vi "JKISM+ State Machine Steps Executed on Sub-Module.vi"() -> ()   [LabVIEW 2014]
uses:
  user.lib/_NEVSTOP/JKI State Machine ++/_Support/JKISMQ/_JKISMQFGV.vi
  user.lib/_NEVSTOP/JKI State Machine ++/JKI-State-Machine-Plus.lvlib
panel:
  in  "Exit":bool
  in  "Run":bool
  out "State History of Sub-Module":string
  out "State History of Main":string
  # "SM: Step1\nSM: Step2 @ Sub-Module\nSM: Step3\nSM: Step4 @ Sub-Module\nSM: Event Check"
  # "(back to step1)"
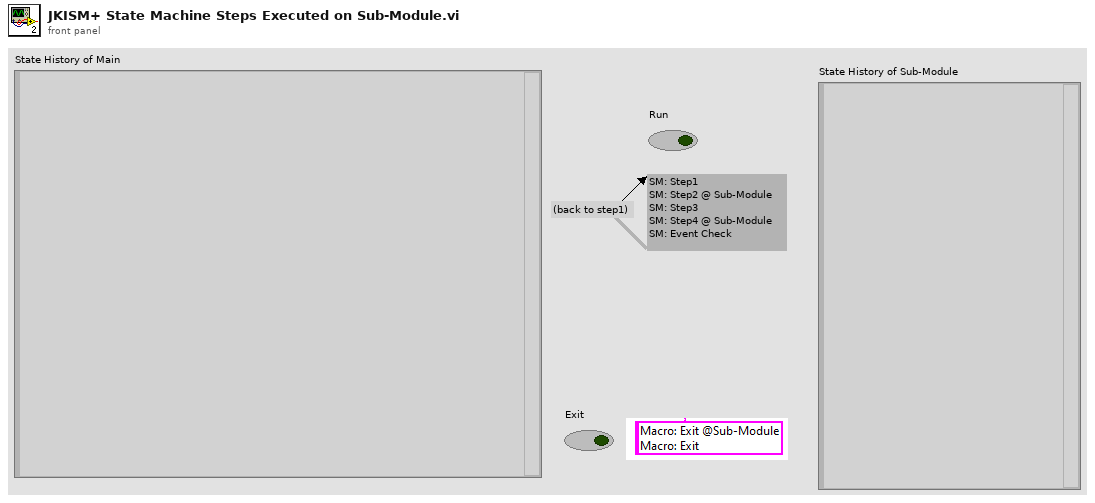
[diagram p1: front panel]
types:
  T1 = enum32{"Invalid", "Standard", "Closed", "Hidden", "Minimized", "Maximized"}
  T2 = enum32{"invalid app kind", "Development System", "Run Time System", "Student Edition", "Embedded LabVIEW", "Evaluation", "Custom"}
  T3 = cluster{"Core":cluster{"Current VI Reference":refnum<vi>, "Close Panel on Exit?":bool}, "Your Boolean data":bool, "State":string}
  T4 = cluster{"Current VI Reference":refnum<vi>, "Close Panel on Exit?":bool}
  T5 = cluster{"Core":cluster{"Current VI Reference":refnum<vi>, "Close Panel on Exit?":bool}, "Your Boolean data":bool, "Your string data":string}
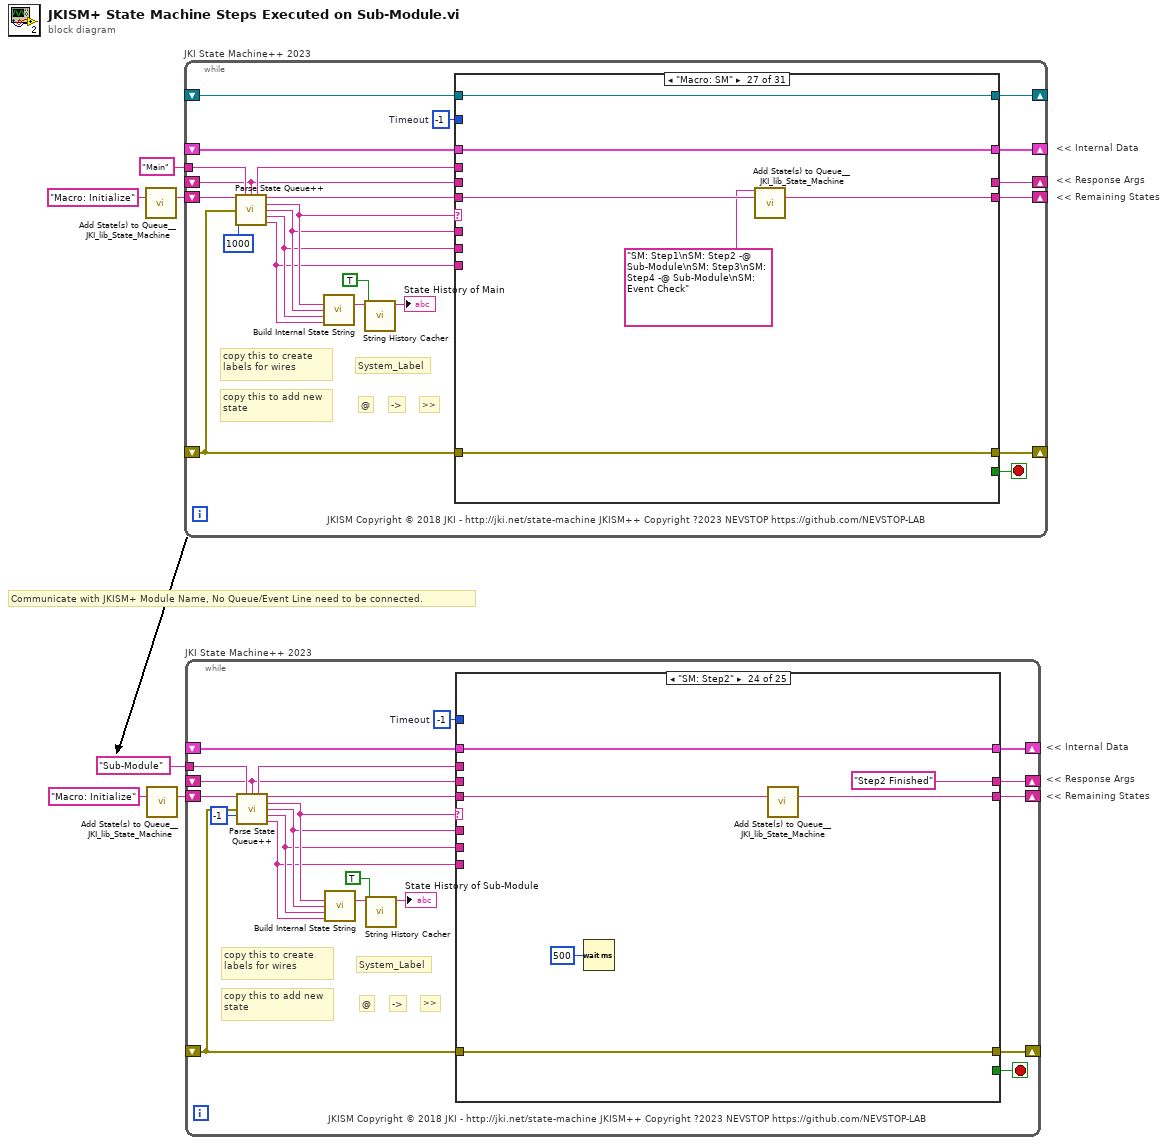
[diagram p0: block diagram]
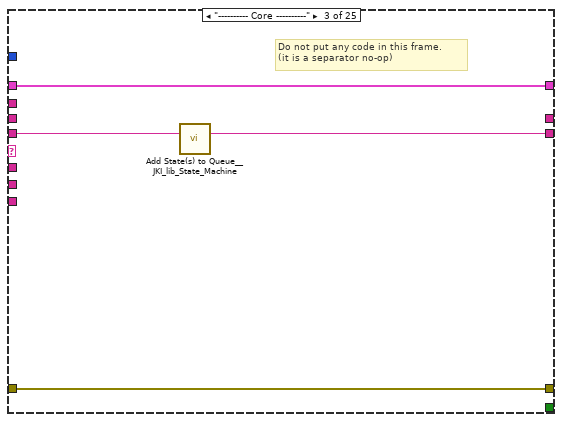
[diagram p4: hidden frame]
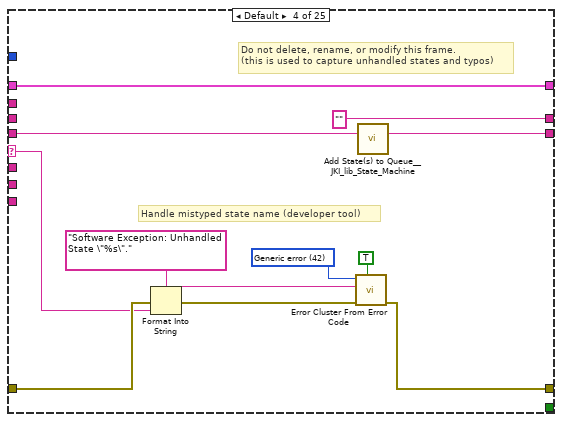
[diagram p5: hidden frame]
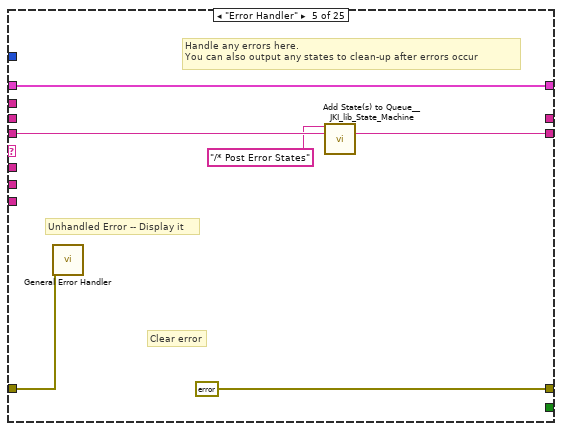
[diagram p6: hidden frame]
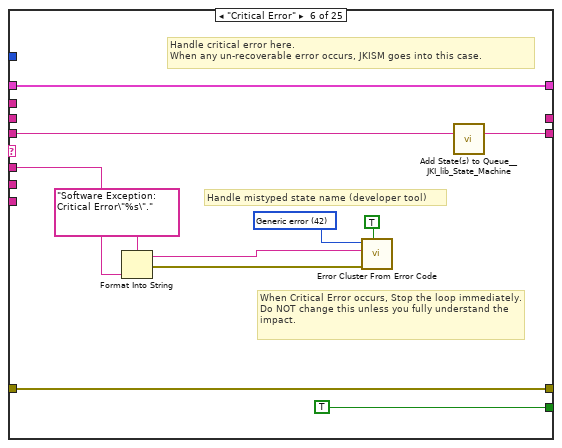
[diagram p7: hidden frame]
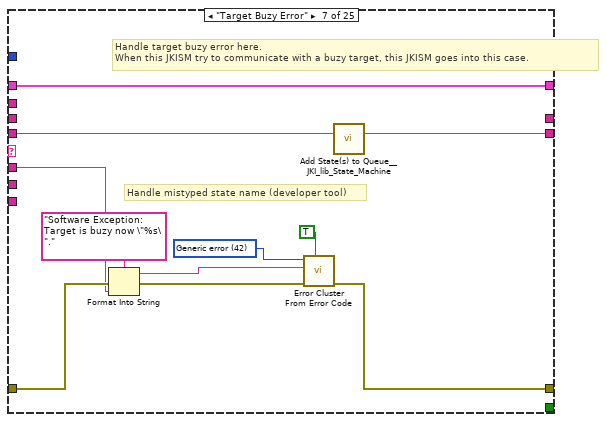
[diagram p8: hidden frame]
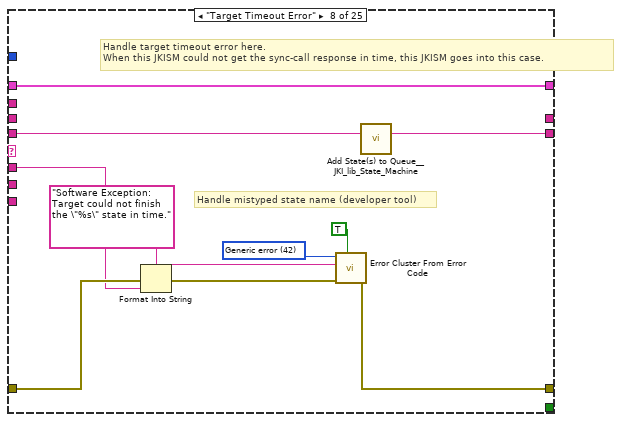
[diagram p9: hidden frame]
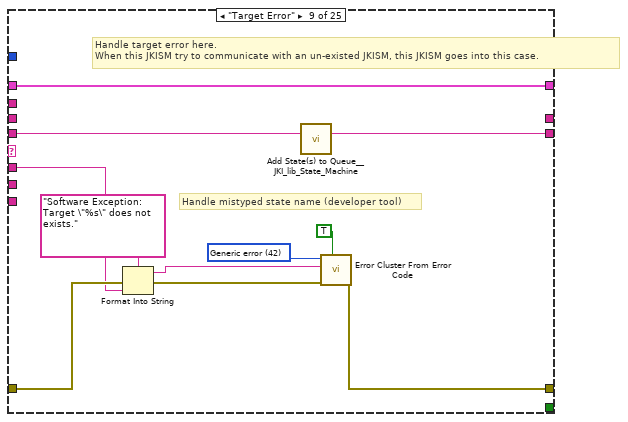
[diagram p10: hidden frame]
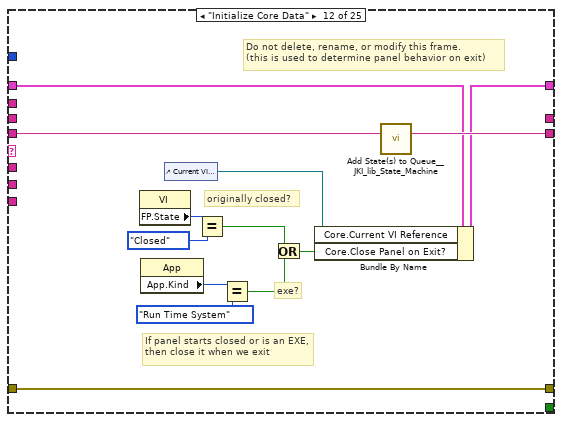
[diagram p13: hidden frame]
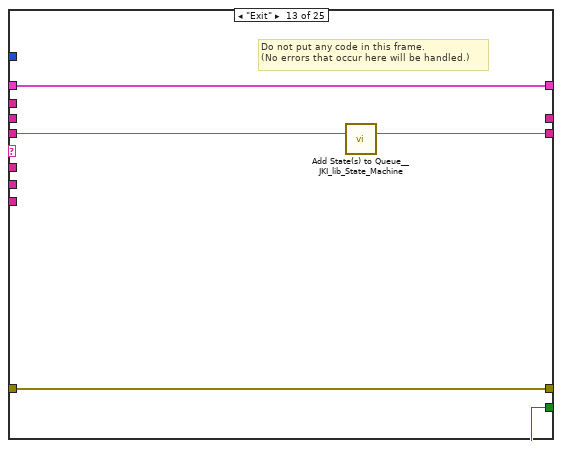
[diagram p14: hidden frame]
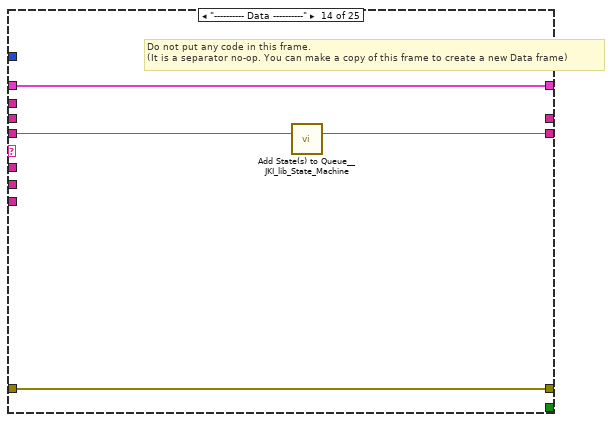
[diagram p15: hidden frame]
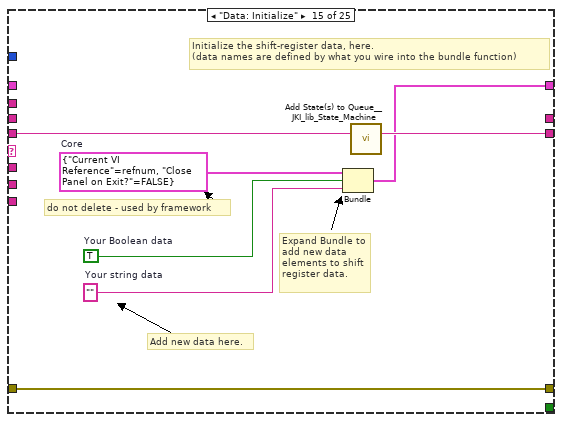
[diagram p16: hidden frame]
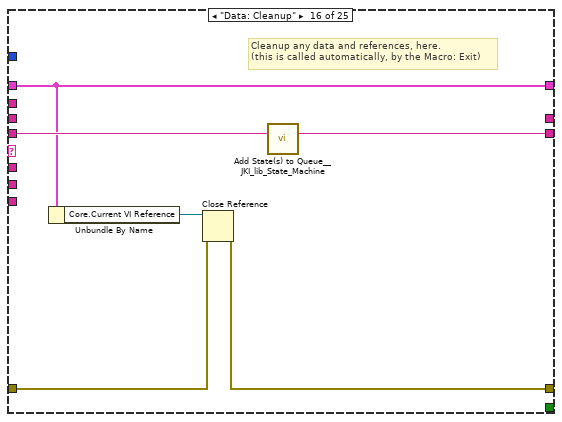
[diagram p17: hidden frame]
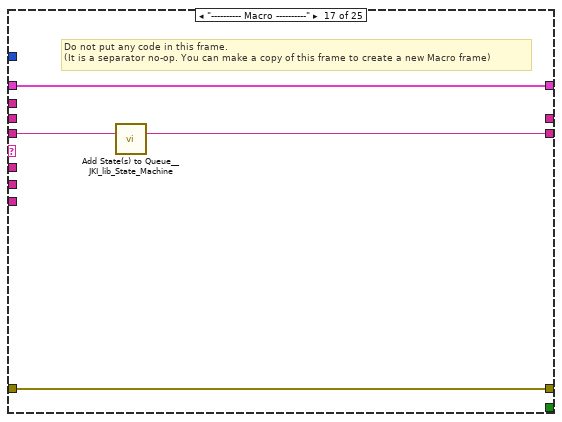
[diagram p18: hidden frame]
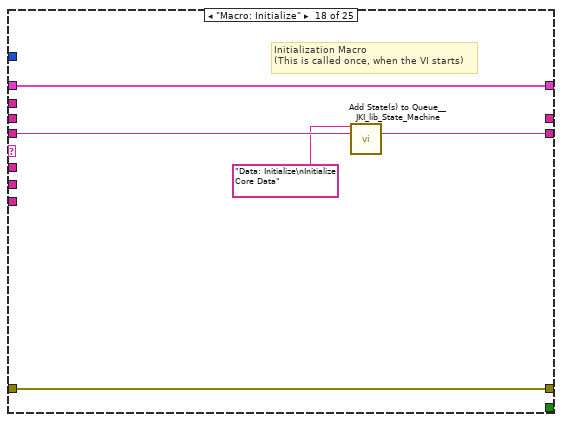
[diagram p19: hidden frame]
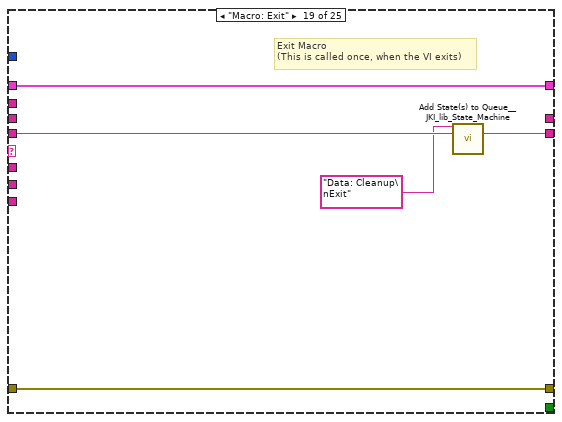
[diagram p20: hidden frame]
diagram:
  # "Communicate with JKISM+ Module Name, No Queue/Event Line need to be connected."
  # "<< Internal Data"
  # "<< Response Args"
  # "<< Remaining States"
  # "<< Internal Data"
  # "<< Response Args"
  # "<< Remaining States"
  n1 = call <vilib>:"Add State(s) to Queue__JKI_lib_State_Machine.vi"("State(s) in (\"\")"="Macro: Initialize") -> ("States Out"=w6:string)  [unwired: 14 in]
  n2 = call <vilib>:"Add State(s) to Queue__JKI_lib_State_Machine.vi"("State(s) in (\"\")"="Macro: Initialize") -> ("States Out"=w1:string)  [unwired: 14 in]
  n3 = while "JKI State Machine++ 2023" {
    shift-right: [w7] -> _
    shift-left: _ -> [w24]
    shift-right: [w27] -> _
    shift-left: _ -> [w22]
    shift-right: [w26] -> _
    shift-left: w6 -> [w28]
    tunnel: "Main" ("Name(\"\" to use uuid)") -> [w17]
    shift-right: [w20] -> _
    shift-left: _ -> [w9]
    shift-right: [w19] -> _
    shift-left: _ -> [w18]
    stop <- w25 stop-if-true
    w23 = -1  # Timeout
    # "JKISM Copyright © 2018 JKI - http://jki.net/state-machine JKISM++ Copyright ?2023 NEVSTOP https://github.com/NEVSTOP-LAB"
    # "copy this to add new state"
    # ">>"
    # "->"
    # "@"
    # "copy this to create labels for wires"
    # "System_Label"
    n4 = call "Parse State Queue++.vi"("State Queue"=w28, "Name(\"\" to use uuid)"=w17, "Response Arguments"=w9, "Error In (no error)"=w22, "Response Timeout(5000ms)"=1000 ("Response Timeout(1000ms)")) -> ("Name Used"=w10:string, "Remaining States"=w29:string, "Current State"=w14:string, "Arguments"=w13:string, "Argument - State"=w12:string, "From Who"=w11:string)  [unwired: 5 in]
    n5 = call "Build Internal State String.vi"("State"=w14, "Arguments (\"\")"=w13, "Arg-State (\"\")"=w12, "Source (\"\")"=w11) -> ("State with Arguments"=w15:string)  [unwired: 11 in]
    n6 = call "String History Cacher.vi"("Include Timestamp(F)"=TRUE, "String"=w15) -> ("String Cache"=→"State History of Main":string)  [unwired: 9 in]
    n7 = case shown="\"Macro: SM\"" w14 {
      selector: w14 -> [_ _ _ w74 _ _ _ _ _ _ _ _ _ _ _ _ _ _ _ _ _ _ _ _ _ _ _ _ _ _ _]
      tunnel: w29 -> [w32 w65 w71 w78 w91 w101 w104 w121 w133 w142 w146 w161 w167 w172 w180 w187 w192 w198 w202 w208 w214 w221 w233 w303 w309 w320 w323 w329 w335 w341 w349]
      tunnel: w13 -> [_ _ _ _ _ w94 w106 w117 w129 _ _ _ _ _ _ _ _ _ _ _ _ w216 w227 _ _ _ _ _ _ _ _]
      tunnel: w24 -> [w37 w64 w68 w76 w88 w102 w108 w119 w131 w141 w145 w154 w165 w169 _ w182 w189 w197 w201 w205 w212 w219 w229 w300 w306 w317 w325 w328 w334 w340 w351]
      tunnel: [w36 w66 w69 w80 errorcluster {"status"=FALSE, "code"=0, "source"=""} ("error out") w103 w111 w123 w135 w143 w147 w158 w164 w170 w177 w183 w190 w193 w200 w206 w211 w217 w230 w301 w307 w318 w326 w330 w336 w342 w352] -> w27
      tunnel: w22 -> [w35 w66 w69 w79 w87 w103 w110 w122 w134 w143 w147 w158 w164 w170 w177 w184 w190 _ w203 w206 w211 w218 w231 w301 w307 w318 w326 w330 w336 w342 w352]
      tunnel: [w38 w65 w70 w77 w90 w100 w109 w120 w132 w142 w146 w160 w166 w171 w179 w186 w191 w198 w202 w207 w213 w220 w232 w302 w308 w319 w322 w329 w335 w341 w348] -> w26
      tunnel: [_ _ _ _ _ TRUE _ _ _ _ _ _ TRUE _ _ _ _ _ _ _ _ _ _ _ _ _ _ _ _ _ _] -> w25
      tunnel: [w34 w64 w68 w76 w88 w102 w108 w119 w131 w141 w145 w159 w165 w169 w178 w182 w189 w197 w201 w205 w212 w219 w229 w300 w306 w317 w325 w328 w334 w340 w351] -> w7
      tunnel: w23 -> [w31 _ _ _ _ _ _ _ _ _ _ _ _ _ _ _ _ _ _ _ _ _ _ _ _ _ _ _ _ _ _]
      tunnel: w11 -> [_ _ _ _ _ _ _ _ _ _ _ _ _ _ _ _ _ _ _ _ _ _ _ _ _ _ _ _ _ _ _]
      tunnel: w12 -> [_ _ _ _ _ _ _ _ _ _ _ _ _ _ _ _ _ _ _ _ _ _ _ _ _ _ _ _ _ _ _]
      tunnel: [_ _ _ "" _ _ _ _ _ _ _ _ _ _ _ _ _ _ _ _ _ _ _ _ _ _ _ _ "Step1 Finished" "Step3 Finished" _] -> w20
      tunnel: [w33 w63 w67 w72 w85 w92 w105 w116 w128 w140 w144 w148 w162 w168 w173 w181 w188 w196 w199 w204 w210 w215 w226 w299 w304 w310 w324 w327 w333 w339 w350] -> w19
      tunnel: w18 -> [w33 w63 w67 w72 w85 w92 w105 w116 w128 w140 w144 w148 w162 w168 w173 w181 w188 _ w199 w204 w210 w215 w226 w299 w304 w310 w324 w327 w333 w339 w350]
      tunnel: w10 -> [_ _ _ _ _ _ _ _ _ _ _ _ _ _ _ _ _ w195 _ _ _ _ _ _ _ _ _ _ _ _ _]
      tunnel: w9 -> [_ _ _ _ _ _ _ _ _ _ _ _ _ _ _ _ _ _ _ _ _ _ _ _ _ _ _ _ _ _ _]
      frame "", "Event Structure", "Idle" {
        # "executes when the state queue is empty"
        n8 = call "Timeout Selector.vi"("Remaining States"=w32, "Timeout Expected"=w31) -> ("Timeout"=w30:i32)  [unwired: 5 in]
        n9 = event shown="[2] \"Run\": Value Change" {
          selector: w33 -> [_ _ _ _ _]
          dyn-events: _ -> [_ _ _ _ _]
          timeout: w30 -> [_ _ _ _ _]
          tunnel: w32 -> [w42 w44 w48 w57 w62]
          tunnel: [w41 w44 w49 w56 w61] -> w38
          tunnel: w37 -> [w39 w45 w50 w54 w59]
          tunnel: [w40 w43 w51 w55 w60] -> w36
          tunnel: w35 -> [w40 w43 w51 w55 w60]
          tunnel: [w39 w45 w50 w54 w59] -> w34
          event Timeout {
            n10 = event-data() -> ()  [unwired: 1 in, 1 out]
            n11 = call <vilib>:"Add State(s) to Queue__JKI_lib_State_Machine.vi"("State(s) in (\"\")"=w42) -> ("States Out"=w41:string)  [unwired: 14 in]
          }
          event User Event {
            # "This user event is used to break out JKISM from waiting in the event structure, to process the next state from external. DO NOT place any code here unless you really need to."
            n12 = event-data() -> ()  [unwired: 1 in, 1 out]
          }
          event "Run": Value Change {
            n13 = event-data() -> ("NewVal"=w47:bool)  [unwired: 1 in]
            n14 = call "Add State(s) to Queue By BOOL(Element).vi"("TRUE(Empty)"="Macro: SM", "Bool"=w47, "Remaining States"=w48) -> ("States Out"=w49:string)  [unwired: 8 in]
          }
          event Panel Close? {
            # "Discard the event because we'll close the front panel ourselves in Macro: Exit"
            # "Close Panel button (pressed) Event\n(this executes Macro: Exit to terminate the VI)"
            n15 = event-data() -> ()  [unwired: 1 in, 1 out]
            n16 = call <vilib>:"Add State(s) to Queue__JKI_lib_State_Machine.vi"("State(s) in Front (\"\")"="Macro: Exit @ Message Handler\nMacro: Exit", "State(s) in (\"\")"=w57) -> ("States Out"=w56:string)  [unwired: 13 in]
            n17 = event-data("Discard?"=TRUE) -> ()  [unwired: 1 in, 1 out]
          }
          event "Exit": Value Change {
            # "Close Panel button (pressed) Event\n(this executes Macro: Exit to terminate the VI)"
            n18 = event-data() -> ()  [unwired: 1 in, 6 out]
            n19 = call <vilib>:"Add State(s) to Queue__JKI_lib_State_Machine.vi"("State(s) in Front (\"\")"="Macro: Exit -@Sub-Module\nMacro: Exit", "State(s) in (\"\")"=w62) -> ("States Out"=w61:string)  [unwired: 13 in]
          }
        }
      }
      frame "JKISM++ Documentation" {
        # "Commenting:\nTo add a comment use \"//\" or \"#\" and all text to the right will be ignored\nCommenting Example:\nUI: Initialize // This initializes the UI\n# This whole line is a comment\n// Another comment line"
        # "State Syntax:\nStateCategory: State >> Argument @ JKISMName\nStateCategory: State >> Argument -> JKISMName\n\nLine Terminator: Line feed"
        # "JKISM++ Documentation"
      }
      frame "---------- Core ----------" {
        # "Do not put any code in this frame.\n(it is a separator no-op)"
        n20 = call <vilib>:"Add State(s) to Queue__JKI_lib_State_Machine.vi"("State(s) in (\"\")"=w71) -> ("States Out"=w70:string)  [unwired: 14 in]
      }
      frame Default {
        w83 = 42 items=["No error", "Argument error", "Memory is full", "Out of zone", "End of file", "File already open", "Generic file I/O error", "File not found", "File permission error", "Disk is full", "Duplicate path", "Too many files open", "System feature not enabled", "Resource file not found", "Cannot add resource", "Resource not found", "Image not found", "Image memory error", "Pen does not exist", "Config type invalid", "Config token not found", "Config parse error", "Config memory error", "Bad external code format", "Bad external code offset", "External code not present", "Null window", "Destroy window error", "Null menu", "Print aborted", "Bad print record", "Print driver error", "Windows error during printing", "Memory error during printing", "Print dialog error", "Generic print error", "Invalid device refnum", "Device not found", "Device parameter error", "Device unit error", "Cannot open device", "Device call aborted", "Generic error", "Cancelled by user", "Object ID too low", "Object ID too high", "Object not in heap", "Unknown heap", "Unknown object (invalid DefProc)", "Unknown object (DefProc not in table)", "Message out of range", "Invalid (null) method", "Unknown message", "Manager call not supported", "Bad address", "Network operation in progress", "Network operation timed out", "Connection is busy", "Network attribute not supported", "Network error", "Address in use", "System out of memory", "Connection aborted", "Connection refused", "Not connected", "Already connected", "Connection closed", "Initialization error (interapplication manager)", "Bad occurrence", "Wait on unbound occurrence handler", "Occurrence queue overflow", "Datalog type conflict", "Unused", "Unrecognized type (interapplication manager)", "Memory corrupt", "Failed to make temporary DLL", "Old CIN version", "Drag socket not found", "Failed to load drop-object", "Failed to register OLE object", "Failed to release OLE object", "Format specifier type mismatch", "Unknown format specifier", "Too few format specifiers", "Too many format specifiers", "Scan failed", "Newer CIN version", "Error converting to variant", "Runtime menu error", "Password tampered", "Variant attribute not found", "Incompatible variant data type", "Event data is not available", "Event Store is not present", "Occurrence is not found", "Event Queue is not created", "Event info is not available", "Refnum passed is NULL", "Error retrieving Class GUID", "Error retrieving CoClass GUID", "Error retrieving TypeLib GUID.", "Bad built application magic bytes.", "Specific driver is different from the specific driver associated with the Logical Name.", "There is no session opened to the class driver.", "Max Error", "MAX - Error with config objects", "MAX - Error loading configuration", "MAX - Group not supported"]
        # "Do not delete, rename, or modify this frame.\n(this is used to capture unhandled states and typos)"
        # "Handle mistyped state name (developer tool)"
        n21 = Format Into String(format string="Software Exception: Unhandled State \"%s\"." ("message"), error in=w79, w74) -> (resulting string=w82:string, error out=w81:errorcluster)  [unwired: 1 in]
        n22 = call <vilib>:"Error Cluster From Error Code.vi"("show call chain? (False)"=TRUE, "error in (no error)"=w81, "error message (\"\")"=w82, "error code (0)"=w83) -> ("error out"=w80:errorcluster)  [unwired: 5 in]
        n23 = call <vilib>:"Add State(s) to Queue__JKI_lib_State_Machine.vi"("State(s) in (\"\")"=w78) -> ("States Out"=w77:string)  [unwired: 14 in]
      }
      frame "Error Handler" {
        # "Unhandled Error -- Display it"
        # "Handle any errors here.\nYou can also output any states to clean-up after errors occur"
        # "Clear error"
        n24 = call <vilib>:"General Error Handler.vi"("error in (no error)"=w87) -> ()  [unwired: 10 in, 5 out]
        n25 = call <vilib>:"Add State(s) to Queue__JKI_lib_State_Machine.vi"("State(s) in Front (\"\")"="/* Post Error States", "State(s) in (\"\")"=w91) -> ("States Out"=w90:string)  [unwired: 13 in]
      }
      frame "Critical Error" {
        w98 = 42 items=["No error", "Argument error", "Memory is full", "Out of zone", "End of file", "File already open", "Generic file I/O error", "File not found", "File permission error", "Disk is full", "Duplicate path", "Too many files open", "System feature not enabled", "Resource file not found", "Cannot add resource", "Resource not found", "Image not found", "Image memory error", "Pen does not exist", "Config type invalid", "Config token not found", "Config parse error", "Config memory error", "Bad external code format", "Bad external code offset", "External code not present", "Null window", "Destroy window error", "Null menu", "Print aborted", "Bad print record", "Print driver error", "Windows error during printing", "Memory error during printing", "Print dialog error", "Generic print error", "Invalid device refnum", "Device not found", "Device parameter error", "Device unit error", "Cannot open device", "Device call aborted", "Generic error", "Cancelled by user", "Object ID too low", "Object ID too high", "Object not in heap", "Unknown heap", "Unknown object (invalid DefProc)", "Unknown object (DefProc not in table)", "Message out of range", "Invalid (null) method", "Unknown message", "Manager call not supported", "Bad address", "Network operation in progress", "Network operation timed out", "Connection is busy", "Network attribute not supported", "Network error", "Address in use", "System out of memory", "Connection aborted", "Connection refused", "Not connected", "Already connected", "Connection closed", "Initialization error (interapplication manager)", "Bad occurrence", "Wait on unbound occurrence handler", "Occurrence queue overflow", "Datalog type conflict", "Unused", "Unrecognized type (interapplication manager)", "Memory corrupt", "Failed to make temporary DLL", "Old CIN version", "Drag socket not found", "Failed to load drop-object", "Failed to register OLE object", "Failed to release OLE object", "Format specifier type mismatch", "Unknown format specifier", "Too few format specifiers", "Too many format specifiers", "Scan failed", "Newer CIN version", "Error converting to variant", "Runtime menu error", "Password tampered", "Variant attribute not found", "Incompatible variant data type", "Event data is not available", "Event Store is not present", "Occurrence is not found", "Event Queue is not created", "Event info is not available", "Refnum passed is NULL", "Error retrieving Class GUID", "Error retrieving CoClass GUID", "Error retrieving TypeLib GUID.", "Bad built application magic bytes.", "Specific driver is different from the specific driver associated with the Logical Name.", "There is no session opened to the class driver.", "Max Error", "MAX - Error with config objects", "MAX - Error loading configuration", "MAX - Group not supported"]
        # "Handle critical error here.\nWhen any un-recoverable error occurs, JKISM goes into this case."
        # "When Critical Error occurs, Stop the loop immediately. Do NOT change this unless you fully understand the impact."
        # "Handle mistyped state name (developer tool)"
        n26 = Format Into String(format string="Software Exception: Critical Error\"%s\"." ("message"), w94) -> (resulting string=w97:string, error out=w96:errorcluster)  [unwired: 2 in]
        n27 = call <vilib>:"Error Cluster From Error Code.vi"("show call chain? (False)"=TRUE, "error in (no error)"=w96, "error message (\"\")"=w97, "error code (0)"=w98) -> ()  [unwired: 5 in, 1 out]
        n28 = call <vilib>:"Add State(s) to Queue__JKI_lib_State_Machine.vi"("State(s) in (\"\")"=w101) -> ("States Out"=w100:string)  [unwired: 14 in]
      }
      frame "Target Buzy Error" {
        w114 = 42 items=["No error", "Argument error", "Memory is full", "Out of zone", "End of file", "File already open", "Generic file I/O error", "File not found", "File permission error", "Disk is full", "Duplicate path", "Too many files open", "System feature not enabled", "Resource file not found", "Cannot add resource", "Resource not found", "Image not found", "Image memory error", "Pen does not exist", "Config type invalid", "Config token not found", "Config parse error", "Config memory error", "Bad external code format", "Bad external code offset", "External code not present", "Null window", "Destroy window error", "Null menu", "Print aborted", "Bad print record", "Print driver error", "Windows error during printing", "Memory error during printing", "Print dialog error", "Generic print error", "Invalid device refnum", "Device not found", "Device parameter error", "Device unit error", "Cannot open device", "Device call aborted", "Generic error", "Cancelled by user", "Object ID too low", "Object ID too high", "Object not in heap", "Unknown heap", "Unknown object (invalid DefProc)", "Unknown object (DefProc not in table)", "Message out of range", "Invalid (null) method", "Unknown message", "Manager call not supported", "Bad address", "Network operation in progress", "Network operation timed out", "Connection is busy", "Network attribute not supported", "Network error", "Address in use", "System out of memory", "Connection aborted", "Connection refused", "Not connected", "Already connected", "Connection closed", "Initialization error (interapplication manager)", "Bad occurrence", "Wait on unbound occurrence handler", "Occurrence queue overflow", "Datalog type conflict", "Unused", "Unrecognized type (interapplication manager)", "Memory corrupt", "Failed to make temporary DLL", "Old CIN version", "Drag socket not found", "Failed to load drop-object", "Failed to register OLE object", "Failed to release OLE object", "Format specifier type mismatch", "Unknown format specifier", "Too few format specifiers", "Too many format specifiers", "Scan failed", "Newer CIN version", "Error converting to variant", "Runtime menu error", "Password tampered", "Variant attribute not found", "Incompatible variant data type", "Event data is not available", "Event Store is not present", "Occurrence is not found", "Event Queue is not created", "Event info is not available", "Refnum passed is NULL", "Error retrieving Class GUID", "Error retrieving CoClass GUID", "Error retrieving TypeLib GUID.", "Bad built application magic bytes.", "Specific driver is different from the specific driver associated with the Logical Name.", "There is no session opened to the class driver.", "Max Error", "MAX - Error with config objects", "MAX - Error loading configuration", "MAX - Group not supported"]
        # "Handle target buzy error here.\nWhen this JKISM try to communicate with a buzy target, this JKISM goes into this case."
        # "Handle mistyped state name (developer tool)"
        n29 = Format Into String(format string="Software Exception: Target is buzy now \"%s\"." ("message"), error in=w110, w106) -> (resulting string=w113:string, error out=w112:errorcluster)  [unwired: 1 in]
        n30 = call <vilib>:"Error Cluster From Error Code.vi"("show call chain? (False)"=TRUE, "error in (no error)"=w112, "error message (\"\")"=w113, "error code (0)"=w114) -> ("error out"=w111:errorcluster)  [unwired: 5 in]
        n31 = call <vilib>:"Add State(s) to Queue__JKI_lib_State_Machine.vi"("State(s) in (\"\")"=w104) -> ("States Out"=w109:string)  [unwired: 14 in]
      }
      frame "Target Timeout Error" {
        w126 = 42 items=["No error", "Argument error", "Memory is full", "Out of zone", "End of file", "File already open", "Generic file I/O error", "File not found", "File permission error", "Disk is full", "Duplicate path", "Too many files open", "System feature not enabled", "Resource file not found", "Cannot add resource", "Resource not found", "Image not found", "Image memory error", "Pen does not exist", "Config type invalid", "Config token not found", "Config parse error", "Config memory error", "Bad external code format", "Bad external code offset", "External code not present", "Null window", "Destroy window error", "Null menu", "Print aborted", "Bad print record", "Print driver error", "Windows error during printing", "Memory error during printing", "Print dialog error", "Generic print error", "Invalid device refnum", "Device not found", "Device parameter error", "Device unit error", "Cannot open device", "Device call aborted", "Generic error", "Cancelled by user", "Object ID too low", "Object ID too high", "Object not in heap", "Unknown heap", "Unknown object (invalid DefProc)", "Unknown object (DefProc not in table)", "Message out of range", "Invalid (null) method", "Unknown message", "Manager call not supported", "Bad address", "Network operation in progress", "Network operation timed out", "Connection is busy", "Network attribute not supported", "Network error", "Address in use", "System out of memory", "Connection aborted", "Connection refused", "Not connected", "Already connected", "Connection closed", "Initialization error (interapplication manager)", "Bad occurrence", "Wait on unbound occurrence handler", "Occurrence queue overflow", "Datalog type conflict", "Unused", "Unrecognized type (interapplication manager)", "Memory corrupt", "Failed to make temporary DLL", "Old CIN version", "Drag socket not found", "Failed to load drop-object", "Failed to register OLE object", "Failed to release OLE object", "Format specifier type mismatch", "Unknown format specifier", "Too few format specifiers", "Too many format specifiers", "Scan failed", "Newer CIN version", "Error converting to variant", "Runtime menu error", "Password tampered", "Variant attribute not found", "Incompatible variant data type", "Event data is not available", "Event Store is not present", "Occurrence is not found", "Event Queue is not created", "Event info is not available", "Refnum passed is NULL", "Error retrieving Class GUID", "Error retrieving CoClass GUID", "Error retrieving TypeLib GUID.", "Bad built application magic bytes.", "Specific driver is different from the specific driver associated with the Logical Name.", "There is no session opened to the class driver.", "Max Error", "MAX - Error with config objects", "MAX - Error loading configuration", "MAX - Group not supported"]
        # "Handle target timeout error here.\nWhen this JKISM could not get the sync-call response in time, this JKISM goes into this case."
        # "Handle mistyped state name (developer tool)"
        n32 = Format Into String(format string="Software Exception: Target could not finish the \"%s\" state in time." ("message"), error in=w122, w117) -> (resulting string=w125:string, error out=w124:errorcluster)  [unwired: 1 in]
        n33 = call <vilib>:"Error Cluster From Error Code.vi"("show call chain? (False)"=TRUE, "error in (no error)"=w124, "error message (\"\")"=w125, "error code (0)"=w126) -> ("error out"=w123:errorcluster)  [unwired: 5 in]
        n34 = call <vilib>:"Add State(s) to Queue__JKI_lib_State_Machine.vi"("State(s) in (\"\")"=w121) -> ("States Out"=w120:string)  [unwired: 14 in]
      }
      frame "Target Error" {
        w138 = 42 items=["No error", "Argument error", "Memory is full", "Out of zone", "End of file", "File already open", "Generic file I/O error", "File not found", "File permission error", "Disk is full", "Duplicate path", "Too many files open", "System feature not enabled", "Resource file not found", "Cannot add resource", "Resource not found", "Image not found", "Image memory error", "Pen does not exist", "Config type invalid", "Config token not found", "Config parse error", "Config memory error", "Bad external code format", "Bad external code offset", "External code not present", "Null window", "Destroy window error", "Null menu", "Print aborted", "Bad print record", "Print driver error", "Windows error during printing", "Memory error during printing", "Print dialog error", "Generic print error", "Invalid device refnum", "Device not found", "Device parameter error", "Device unit error", "Cannot open device", "Device call aborted", "Generic error", "Cancelled by user", "Object ID too low", "Object ID too high", "Object not in heap", "Unknown heap", "Unknown object (invalid DefProc)", "Unknown object (DefProc not in table)", "Message out of range", "Invalid (null) method", "Unknown message", "Manager call not supported", "Bad address", "Network operation in progress", "Network operation timed out", "Connection is busy", "Network attribute not supported", "Network error", "Address in use", "System out of memory", "Connection aborted", "Connection refused", "Not connected", "Already connected", "Connection closed", "Initialization error (interapplication manager)", "Bad occurrence", "Wait on unbound occurrence handler", "Occurrence queue overflow", "Datalog type conflict", "Unused", "Unrecognized type (interapplication manager)", "Memory corrupt", "Failed to make temporary DLL", "Old CIN version", "Drag socket not found", "Failed to load drop-object", "Failed to register OLE object", "Failed to release OLE object", "Format specifier type mismatch", "Unknown format specifier", "Too few format specifiers", "Too many format specifiers", "Scan failed", "Newer CIN version", "Error converting to variant", "Runtime menu error", "Password tampered", "Variant attribute not found", "Incompatible variant data type", "Event data is not available", "Event Store is not present", "Occurrence is not found", "Event Queue is not created", "Event info is not available", "Refnum passed is NULL", "Error retrieving Class GUID", "Error retrieving CoClass GUID", "Error retrieving TypeLib GUID.", "Bad built application magic bytes.", "Specific driver is different from the specific driver associated with the Logical Name.", "There is no session opened to the class driver.", "Max Error", "MAX - Error with config objects", "MAX - Error loading configuration", "MAX - Group not supported"]
        # "Handle target error here.\nWhen this JKISM try to communicate with an un-existed JKISM, this JKISM goes into this case."
        # "Handle mistyped state name (developer tool)"
        n35 = Format Into String(format string="Software Exception: Target \"%s\" does not exists." ("message"), error in=w134, w129) -> (resulting string=w137:string, error out=w136:errorcluster)  [unwired: 1 in]
        n36 = call <vilib>:"Add State(s) to Queue__JKI_lib_State_Machine.vi"("State(s) in (\"\")"=w133) -> ("States Out"=w132:string)  [unwired: 14 in]
        n37 = call <vilib>:"Error Cluster From Error Code.vi"("show call chain? (False)"=TRUE, "error in (no error)"=w136, "error message (\"\")"=w137, "error code (0)"=w138) -> ("error out"=w135:errorcluster)  [unwired: 5 in]
      }
      frame "Async Response", "Response" {
        # "Handle Async-call Response (\"Async Response\" for ->)"
        # "Handle Sync-call Response (\"Response\" for @)"
        # "After Message is excuted, JKISM+ goes to this state for recieve the response. \n    For Async Message(->), \"Async Response\" is used. This JKISM will goes to \"Async Message Posted\" immediately and recieve the \"Async Response\" after the callee finishes the message.\n    For Sync Message(@),  This JKISM will wait until the message is done and immidieatly goes to \"Response\""
      }
      frame "Async Message Posted" {
        # "Handle post action for async message (->)."
        # "After Async Message is posted (->), JKISM+ goes to this state for post-action. You can use Argument - State to tell which Async Message is called."
      }
      frame "Initialize Core Data" {
        # "Do not delete, rename, or modify this frame.\n(this is used to determine panel behavior on exit)"
        # "originally closed?"
        # "exe?"
        # "If panel starts closed or is an EXE, then close it when we exit"
        n38 = property class="VI"() -> ("FP.State"=w151:T1)  [unwired: 2 in, 2 out]
        n39 = property class="App"() -> ("App.Kind"=w157:T2)  [unwired: 2 in, 2 out]
        n40 = control-ref of="Current VI Reference"() -> (w152:refnum<vi>)
        n41 = Equal?(x=w151, y=T1."Closed" ("Front Panel Window:State")) -> (x = y?=w149:bool)
        n42 = Equal?(x=w157, y=T2."Run Time System" ("Application:Kind")) -> (x = y?=w155:bool)
        n43 = Or(x=w149, y=w155) -> (x .or. y?=w153:bool)
        n44 = Bundle By Name(cluster=w154, "Core.Current VI Reference"=w152, "Core.Close Panel on Exit?"=w153) -> (w159:T3)
        n45 = call <vilib>:"Add State(s) to Queue__JKI_lib_State_Machine.vi"("State(s) in (\"\")"=w161) -> ("States Out"=w160:string)  [unwired: 14 in]
      }
      frame "Exit" {
        # "Do not put any code in this frame.\n(No errors that occur here will be handled.)"
        n46 = call <vilib>:"Add State(s) to Queue__JKI_lib_State_Machine.vi"("State(s) in (\"\")"=w167) -> ("States Out"=w166:string)  [unwired: 14 in]
      }
      frame "---------- Data ----------" {
        # "Do not put any code in this frame.\n(It is a separator no-op. You can make a copy of this frame to create a new Data frame)"
        n47 = call <vilib>:"Add State(s) to Queue__JKI_lib_State_Machine.vi"("State(s) in (\"\")"=w172) -> ("States Out"=w171:string)  [unwired: 14 in]
      }
      frame "Data: Initialize" {
        w174 = T4 {"Current VI Reference"=refnum, "Close Panel on Exit?"=FALSE}  # Core
        w176 = TRUE  # Your Boolean data
        w175 = ""  # State
        # "do not delete - used by framework"
        # "Initialize the shift-register data, here.\n(data names are defined by what you wire into the bundle function)"
        n48 = Bundle("Core"=w174, "Your Boolean data"=w176, "State"=w175) -> (w178:T3)  [unwired: 1 in]
        n49 = call <vilib>:"Add State(s) to Queue__JKI_lib_State_Machine.vi"("State(s) in (\"\")"=w180) -> ("States Out"=w179:string)  [unwired: 14 in]
      }
      frame "Data: Cleanup" {
        # "Cleanup any data and references, here.\n(this is called automatically, by the Macro: Exit)"
        n50 = Unbundle By Name(w182) -> ("Core.Current VI Reference"=w185:refnum<vi>)
        n51 = Close Reference(reference=w185, error in (no error)=w184) -> (error out=w183:errorcluster)
        n52 = call <vilib>:"Add State(s) to Queue__JKI_lib_State_Machine.vi"("State(s) in (\"\")"=w187) -> ("States Out"=w186:string)  [unwired: 14 in]
      }
      frame "---------- Events ----------" {
        # "Do not put any code in this frame.\n(It is a separator no-op. You can make a copy of this frame to create a new UI frame)"
        n53 = call <vilib>:"Add State(s) to Queue__JKI_lib_State_Machine.vi"("State(s) in (\"\")"=w192) -> ("States Out"=w191:string)  [unwired: 14 in]
      }
      frame "Events: Register" {
        # "Register message event to break Waiting in Event structure."
        n54 = call "JKISM++ Get New State Notifier Event.vi"("Name(\"\" to use uuid) in"=w195) -> ("Error out"=w193:errorcluster, "New State Notifier Event"=w194:refnum<user-event>)  [unwired: 9 in]
        n55 = register-events(w194) -> (reference out=w196:refnum<event-registration>)  [unwired: 2 in, 1 out]
      }
      frame "Events: Unregister" {
        n56 = Unregister For Events(event registration refnum=w199, error in=w203) -> (error out=w200:errorcluster)
      }
      frame "---------- UI ----------" {
        # "Do not put any code in this frame.\n(It is a separator no-op. You can make a copy of this frame to create a new UI frame)"
        n57 = call <vilib>:"Add State(s) to Queue__JKI_lib_State_Machine.vi"("State(s) in (\"\")"=w208) -> ("States Out"=w207:string)  [unwired: 14 in]
      }
      frame "UI: Initialize" {
        # "Initialize the User Interface, here.\n(this is called automatically, by the Macro: Init)"
        n58 = local write "Run"(FALSE ("Run")) -> ()
        n59 = call <vilib>:"Add State(s) to Queue__JKI_lib_State_Machine.vi"("State(s) in (\"\")"=w214) -> ("States Out"=w213:string)  [unwired: 14 in]
      }
      frame "UI: Cursor Set" {
        # "Argument"
        # "Set and Unset Cursor Busy.\n(Usage: \"UI: Cursor Set >> Busy|Idle\")"
        n60 = case shown="\"Idle\", Default" w216 {
          tunnel: w218 -> [w223 w225]
          tunnel: [w222 w224] -> w217
          frame "Idle", Default {
            n61 = call <vilib>:"Unset Busy.vi"("error in (no error)"=w223) -> ("error out"=w222:errorcluster)  [unwired: 10 in]
          }
          frame "Busy" {
            n62 = call <vilib>:"Set Busy.vi"("error in (no error)"=w225) -> ("error out"=w224:errorcluster)  [unwired: 9 in, 1 out]
          }
        }
        n63 = call <vilib>:"Add State(s) to Queue__JKI_lib_State_Machine.vi"("State(s) in (\"\")"=w221) -> ("States Out"=w220:string)  [unwired: 14 in]
      }
      frame "UI: Front Panel State" {
        # "Argument"
        # "Set Front Panel Open or Closed\n(Usage: \"UI: Front Panel State >> Open|Close\")"
        n64 = Unbundle By Name(w229) -> ("Core.Current VI Reference"=w228:refnum<vi>)
        n65 = call <vilib>:"Add State(s) to Queue__JKI_lib_State_Machine.vi"("State(s) in (\"\")"=w233) -> ("States Out"=w232:string)  [unwired: 14 in]
        n66 = case shown="\"Minimize\", \"Minimized\"" w227 {
          tunnel: w231 -> [w239 w254 w265 w278 w291]
          tunnel: [w241 w255 w267 w280 w293] -> w230
          tunnel: w228 -> [w240 w252 w266 w279 w292]
          frame "Open", "Standard", Default {
            w234 = T1."Standard" ("State")
            n67 = property class="VI"(reference=w240, error in=w239) -> (reference out=w237:refnum<vi>, error out=w238:errorcluster, "FP.State"=w236:T1)
            n68 = Not Equal?(x=w236, y=w234) -> (x != y?=w235:bool)
            n69 = case shown="True" w235 {
              tunnel: [w245 w247] -> w241
              tunnel: w238 -> [w244 w247]
              tunnel: w237 -> [w243 _]
              tunnel: w234 -> [w242 _]
              frame True {
                n70 = invoke class="VI" method="FP.Open"(reference=w243, error in=w244, "Activate"=TRUE, "State"=w242) -> (error out=w245:errorcluster)  [unwired: 1 in, 4 out]
              }
              frame False {
              }
            }
          }
          frame "Close", "Closed" {
            n71 = property class="VI"(reference=w252, error in=w254) -> (reference out=w251:refnum<vi>, error out=w253:errorcluster, "FP.State"=w249:T1)
            n72 = Not Equal?(x=w249, y=T1."Closed" ("Front Panel Window:State")) -> (x != y?=w248:bool)
            n73 = case shown="True" w248 {
              tunnel: [w256 w259] -> w255
              tunnel: w253 -> [w256 w258]
              tunnel: w251 -> [_ w257]
              frame False {
              }
              frame True {
                n74 = invoke class="VI" method="FP.Close"(reference=w257, error in=w258) -> (error out=w259:errorcluster)  [unwired: 1 in, 2 out]
              }
            }
          }
          frame "Hidden", "Hide" {
            w260 = T1."Hidden" ("State")
            n75 = property class="VI"(reference=w266, error in=w265) -> (reference out=w263:refnum<vi>, error out=w264:errorcluster, "FP.State"=w262:T1)
            n76 = Not Equal?(x=w262, y=w260) -> (x != y?=w261:bool)
            n77 = case shown="True" w261 {
              tunnel: [w271 w272] -> w267
              tunnel: w264 -> [w270 w272]
              tunnel: w263 -> [w269 _]
              tunnel: w260 -> [w268 _]
              frame True {
                n78 = invoke class="VI" method="FP.Open"(reference=w269, error in=w270, "State"=w268) -> (error out=w271:errorcluster)  [unwired: 2 in, 4 out]
              }
              frame False {
              }
            }
          }
          frame "Minimize", "Minimized" {
            w273 = T1."Minimized" ("State")
            n79 = property class="VI"(reference=w279, error in=w278) -> (reference out=w276:refnum<vi>, error out=w277:errorcluster, "FP.State"=w275:T1)
            n80 = Not Equal?(x=w275, y=w273) -> (x != y?=w274:bool)
            n81 = case shown="True" w274 {
              tunnel: [w284 w285] -> w280
              tunnel: w277 -> [w283 w285]
              tunnel: w276 -> [w282 _]
              tunnel: w273 -> [w281 _]
              frame True {
                n82 = invoke class="VI" method="FP.Open"(reference=w282, error in=w283, "State"=w281) -> (error out=w284:errorcluster)  [unwired: 2 in, 4 out]
              }
              frame False {
              }
            }
          }
          frame "Maximize", "Maximized" {
            w286 = T1."Maximized" ("State")
            n83 = property class="VI"(reference=w292, error in=w291) -> (reference out=w289:refnum<vi>, error out=w290:errorcluster, "FP.State"=w288:T1)
            n84 = Not Equal?(x=w288, y=w286) -> (x != y?=w287:bool)
            n85 = case shown="True" w287 {
              tunnel: [w297 w298] -> w293
              tunnel: w290 -> [w296 w298]
              tunnel: w289 -> [w295 _]
              tunnel: w286 -> [w294 _]
              frame True {
                n86 = invoke class="VI" method="FP.Open"(reference=w295, error in=w296, "State"=w294) -> (error out=w297:errorcluster)  [unwired: 2 in, 4 out]
              }
              frame False {
              }
            }
          }
        }
      }
      frame "---------- Macro ----------" {
        # "Do not put any code in this frame.\n(It is a separator no-op. You can make a copy of this frame to create a new Macro frame)"
        n87 = call <vilib>:"Add State(s) to Queue__JKI_lib_State_Machine.vi"("State(s) in (\"\")"=w303) -> ("States Out"=w302:string)  [unwired: 14 in]
      }
      frame "Macro: Initialize" {
        w305 = "Data: Initialize\nInitialize Core Data\nEvents: Register\nUI: Initialize\nUI: Front Panel State >> Open"  # Data: Initialize Initialize Core Data Events: Register UI: Initialize UI: Front Panel State >> Open
        # "Initialization Macro\n(This is called once, when the VI starts)"
        n88 = call <vilib>:"Add State(s) to Queue__JKI_lib_State_Machine.vi"("State(s) in Front (\"\")"=w305, "State(s) in (\"\")"=w309) -> ("States Out"=w308:string)  [unwired: 13 in]
      }
      frame "Macro: Exit" {
        # "Exit Macro\n(This is called once, when the VI exits)"
        n89 = Unbundle By Name(w317) -> ("Core.Close Panel on Exit?"=w316:bool)
        n90 = Select(t="UI: Front Panel State >> Close", s=w316, f="") -> (s? t:f=w313:string)
        n91 = call <vilib>:"Add State(s) to Queue__JKI_lib_State_Machine.vi"("State(s) in (\"\")"=w313, "State(s) at Back (\"\")"="Data: Cleanup\nEvents: Unregister\nExit") -> ("States Out"=w311:string)  [unwired: 13 in]
        n92 = call <vilib>:"Add State(s) to Queue__JKI_lib_State_Machine.vi"("State(s) in Front (\"\")"=w311, "State(s) in (\"\")"=w320) -> ("States Out"=w319:string)  [unwired: 13 in]
      }
      frame "Macro: SM" {
        n93 = call <vilib>:"Add State(s) to Queue__JKI_lib_State_Machine.vi"("State(s) in Front (\"\")"="SM: Step1\nSM: Step2 -@ Sub-Module\nSM: Step3\nSM: Step4 -@ Sub-Module\nSM: Event Check" ("State(s) in Front (\"\")"), "State(s) in (\"\")"=w323) -> ("States Out"=w322:string)  [unwired: 13 in]
      }
      frame "---State Machine ---" {
      }
      frame "SM: Step1" {
        n94 = Wait (ms)(milliseconds to wait=u32 500) -> ()  [unwired: 1 out]
      }
      frame "SM: Step3" {
        n95 = Wait (ms)(milliseconds to wait=u32 500) -> ()  [unwired: 1 out]
      }
      frame "SM: Event Check" {
        n96 = Wait (ms)(milliseconds to wait=u32 500) -> ()  [unwired: 1 out]
        n97 = call "Add State(s) to Queue By BOOL(Element).vi"("TRUE(Empty)"="Macro: SM", "Bool"="Run", "Remaining States"="Idle" ("State(s) in Front (\"\")")) -> ("States Out"=w346:string)  [unwired: 8 in]
        n98 = call <vilib>:"Add State(s) to Queue__JKI_lib_State_Machine.vi"("State(s) in Front (\"\")"=w346, "State(s) in (\"\")"=w349) -> ("States Out"=w348:string)  [unwired: 13 in]
      }
    }
  }
  n99 = while "JKI State Machine++ 2023" {
    shift-right: [w368] -> _
    shift-left: _ -> [w367]
    shift-right: [w371] -> _
    shift-left: _ -> [w365]
    shift-right: [w370] -> _
    shift-left: w1 -> [w372]
    tunnel: "Sub-Module" ("Name(\"\" to use uuid) 2") -> [w363]
    shift-right: [w364] -> _
    shift-left: _ -> [w355]
    stop <- w369 stop-if-true
    w366 = -1  # Timeout
    # "JKISM Copyright © 2018 JKI - http://jki.net/state-machine JKISM++ Copyright ?2023 NEVSTOP https://github.com/NEVSTOP-LAB"
    # "copy this to add new state"
    # ">>"
    # "->"
    # "@"
    # "copy this to create labels for wires"
    # "System_Label"
    n100 = call "Parse State Queue++.vi"("State Queue"=w372, "Name(\"\" to use uuid)"=w363, "Response Arguments"=w355, "Error In (no error)"=w365, "Dequeue Timeout(0ms)"=-1) -> ("Name Used"=w356:string, "Remaining States"=w373:string, "Current State"=w360:string, "Arguments"=w359:string, "Argument - State"=w358:string, "From Who"=w357:string)  [unwired: 5 in]
    n101 = call "Build Internal State String.vi"("State"=w360, "Arguments (\"\")"=w359, "Arg-State (\"\")"=w358, "Source (\"\")"=w357) -> ("State with Arguments"=w361:string)  [unwired: 11 in]
    n102 = call "String History Cacher.vi"("Include Timestamp(F)"=TRUE, "String"=w361) -> ("String Cache"=→"State History of Sub-Module":string)  [unwired: 9 in]
    n103 = case shown="\"SM: Step2\"" w360 {
      selector: w360 -> [_ _ _ w385 _ _ _ _ _ _ _ _ _ _ _ _ _ _ _ _ _ _ _ _ _]
      tunnel: w373 -> [w375 w378 w383 w389 w401 w410 w413 w428 w439 w447 w450 w464 w469 w473 w480 w486 w490 w495 w500 w502 w506 w511 w518 w524 w530]
      tunnel: w359 -> [_ _ _ _ _ w403 w414 w424 w435 _ _ _ _ _ _ _ _ _ _ _ _ w509 _ _ _]
      tunnel: w367 -> [w376 w377 w380 w387 w398 w411 w416 w426 w437 w446 w449 w457 w467 w470 _ w481 w487 w492 w497 w501 w505 w510 w515 w521 w527]
      tunnel: [w374 w379 w381 w391 errorcluster {"status"=FALSE, "code"=0, "source"=""} ("error out") w412 w419 w430 w441 w448 w451 w461 w466 w471 w477 w482 w488 w493 w498 w503 w507 w512 w516 w522 w528] -> w371
      tunnel: w365 -> [w374 w379 w381 w390 w397 w412 w418 w429 w440 w448 w451 w461 w466 w471 w477 w483 w488 w493 w498 w503 w507 w512 w516 w522 w528]
      tunnel: [w375 w378 w382 w388 w400 w409 w417 w427 w438 w447 w450 w463 w468 w472 w479 w485 w489 w494 w499 w502 w506 w511 w517 w523 w529] -> w370
      tunnel: [_ _ _ _ _ TRUE _ _ _ _ _ _ TRUE _ _ _ _ _ _ _ _ _ _ _ _] -> w369
      tunnel: [w376 w377 w380 w387 w398 w411 w416 w426 w437 w446 w449 w462 w467 w470 w478 w481 w487 w492 w497 w501 w505 w510 w515 w521 w527] -> w368
      tunnel: w366 -> [_ _ _ _ _ _ _ _ _ _ _ _ _ _ _ _ _ _ _ _ _ _ _ _ _]
      tunnel: w357 -> [_ _ _ _ _ _ _ _ _ _ _ _ _ _ _ _ _ _ _ _ _ _ _ _ _]
      tunnel: w358 -> [_ _ _ _ _ _ _ _ _ _ _ _ _ _ _ _ _ _ _ _ _ _ _ _ _]
      tunnel: [_ _ _ "" _ _ _ _ _ _ _ _ _ _ _ _ _ _ _ _ "API1 Response" w508 _ "Step2 Finished" "Step4 Finished"] -> w364
      tunnel: w356 -> [_ _ _ _ _ _ _ _ _ _ _ _ _ _ _ _ _ _ _ _ _ _ _ _ _]
      tunnel: w355 -> [_ _ _ _ _ _ _ _ _ _ _ _ _ _ _ _ _ _ _ _ _ _ _ _ _]
      frame "", "Idle" {
        # "executes when the state queue is empty"
      }
      frame "JKISM++ Documentation" {
        # "Commenting:\nTo add a comment use \"//\" or \"#\" and all text to the right will be ignored\nCommenting Example:\nUI: Initialize // This initializes the UI\n# This whole line is a comment\n// Another comment line"
        # "State Syntax:\nStateCategory: State >> Argument @ JKISMName\nStateCategory: State >> Argument -> JKISMName\n\nLine Terminator: Line feed"
        # "JKISM++ Documentation"
      }
      frame "---------- Core ----------" {
        # "Do not put any code in this frame.\n(it is a separator no-op)"
        n104 = call <vilib>:"Add State(s) to Queue__JKI_lib_State_Machine.vi"("State(s) in (\"\")"=w383) -> ("States Out"=w382:string)  [unwired: 14 in]
      }
      frame Default {
        w394 = 42 items=["No error", "Argument error", "Memory is full", "Out of zone", "End of file", "File already open", "Generic file I/O error", "File not found", "File permission error", "Disk is full", "Duplicate path", "Too many files open", "System feature not enabled", "Resource file not found", "Cannot add resource", "Resource not found", "Image not found", "Image memory error", "Pen does not exist", "Config type invalid", "Config token not found", "Config parse error", "Config memory error", "Bad external code format", "Bad external code offset", "External code not present", "Null window", "Destroy window error", "Null menu", "Print aborted", "Bad print record", "Print driver error", "Windows error during printing", "Memory error during printing", "Print dialog error", "Generic print error", "Invalid device refnum", "Device not found", "Device parameter error", "Device unit error", "Cannot open device", "Device call aborted", "Generic error", "Cancelled by user", "Object ID too low", "Object ID too high", "Object not in heap", "Unknown heap", "Unknown object (invalid DefProc)", "Unknown object (DefProc not in table)", "Message out of range", "Invalid (null) method", "Unknown message", "Manager call not supported", "Bad address", "Network operation in progress", "Network operation timed out", "Connection is busy", "Network attribute not supported", "Network error", "Address in use", "System out of memory", "Connection aborted", "Connection refused", "Not connected", "Already connected", "Connection closed", "Initialization error (interapplication manager)", "Bad occurrence", "Wait on unbound occurrence handler", "Occurrence queue overflow", "Datalog type conflict", "Unused", "Unrecognized type (interapplication manager)", "Memory corrupt", "Failed to make temporary DLL", "Old CIN version", "Drag socket not found", "Failed to load drop-object", "Failed to register OLE object", "Failed to release OLE object", "Format specifier type mismatch", "Unknown format specifier", "Too few format specifiers", "Too many format specifiers", "Scan failed", "Newer CIN version", "Error converting to variant", "Runtime menu error", "Password tampered", "Variant attribute not found", "Incompatible variant data type", "Event data is not available", "Event Store is not present", "Occurrence is not found", "Event Queue is not created", "Event info is not available", "Refnum passed is NULL", "Error retrieving Class GUID", "Error retrieving CoClass GUID", "Error retrieving TypeLib GUID.", "Bad built application magic bytes.", "Specific driver is different from the specific driver associated with the Logical Name.", "There is no session opened to the class driver.", "Max Error", "MAX - Error with config objects", "MAX - Error loading configuration", "MAX - Group not supported"]
        # "Do not delete, rename, or modify this frame.\n(this is used to capture unhandled states and typos)"
        # "Handle mistyped state name (developer tool)"
        n105 = Format Into String(format string="Software Exception: Unhandled State \"%s\"." ("message"), error in=w390, w385) -> (resulting string=w393:string, error out=w392:errorcluster)  [unwired: 1 in]
        n106 = call <vilib>:"Error Cluster From Error Code.vi"("show call chain? (False)"=TRUE, "error in (no error)"=w392, "error message (\"\")"=w393, "error code (0)"=w394) -> ("error out"=w391:errorcluster)  [unwired: 5 in]
        n107 = call <vilib>:"Add State(s) to Queue__JKI_lib_State_Machine.vi"("State(s) in (\"\")"=w389) -> ("States Out"=w388:string)  [unwired: 14 in]
      }
      frame "Error Handler" {
        # "Unhandled Error -- Display it"
        # "Handle any errors here.\nYou can also output any states to clean-up after errors occur"
        # "Clear error"
        n108 = call <vilib>:"General Error Handler.vi"("error in (no error)"=w397) -> ()  [unwired: 10 in, 5 out]
        n109 = call <vilib>:"Add State(s) to Queue__JKI_lib_State_Machine.vi"("State(s) in Front (\"\")"="/* Post Error States", "State(s) in (\"\")"=w401) -> ("States Out"=w400:string)  [unwired: 13 in]
      }
      frame "Critical Error" {
        w407 = 42 items=["No error", "Argument error", "Memory is full", "Out of zone", "End of file", "File already open", "Generic file I/O error", "File not found", "File permission error", "Disk is full", "Duplicate path", "Too many files open", "System feature not enabled", "Resource file not found", "Cannot add resource", "Resource not found", "Image not found", "Image memory error", "Pen does not exist", "Config type invalid", "Config token not found", "Config parse error", "Config memory error", "Bad external code format", "Bad external code offset", "External code not present", "Null window", "Destroy window error", "Null menu", "Print aborted", "Bad print record", "Print driver error", "Windows error during printing", "Memory error during printing", "Print dialog error", "Generic print error", "Invalid device refnum", "Device not found", "Device parameter error", "Device unit error", "Cannot open device", "Device call aborted", "Generic error", "Cancelled by user", "Object ID too low", "Object ID too high", "Object not in heap", "Unknown heap", "Unknown object (invalid DefProc)", "Unknown object (DefProc not in table)", "Message out of range", "Invalid (null) method", "Unknown message", "Manager call not supported", "Bad address", "Network operation in progress", "Network operation timed out", "Connection is busy", "Network attribute not supported", "Network error", "Address in use", "System out of memory", "Connection aborted", "Connection refused", "Not connected", "Already connected", "Connection closed", "Initialization error (interapplication manager)", "Bad occurrence", "Wait on unbound occurrence handler", "Occurrence queue overflow", "Datalog type conflict", "Unused", "Unrecognized type (interapplication manager)", "Memory corrupt", "Failed to make temporary DLL", "Old CIN version", "Drag socket not found", "Failed to load drop-object", "Failed to register OLE object", "Failed to release OLE object", "Format specifier type mismatch", "Unknown format specifier", "Too few format specifiers", "Too many format specifiers", "Scan failed", "Newer CIN version", "Error converting to variant", "Runtime menu error", "Password tampered", "Variant attribute not found", "Incompatible variant data type", "Event data is not available", "Event Store is not present", "Occurrence is not found", "Event Queue is not created", "Event info is not available", "Refnum passed is NULL", "Error retrieving Class GUID", "Error retrieving CoClass GUID", "Error retrieving TypeLib GUID.", "Bad built application magic bytes.", "Specific driver is different from the specific driver associated with the Logical Name.", "There is no session opened to the class driver.", "Max Error", "MAX - Error with config objects", "MAX - Error loading configuration", "MAX - Group not supported"]
        # "Handle critical error here.\nWhen any un-recoverable error occurs, JKISM goes into this case."
        # "When Critical Error occurs, Stop the loop immediately. Do NOT change this unless you fully understand the impact."
        # "Handle mistyped state name (developer tool)"
        n110 = Format Into String(format string="Software Exception: Critical Error\"%s\"." ("message"), w403) -> (resulting string=w406:string, error out=w405:errorcluster)  [unwired: 2 in]
        n111 = call <vilib>:"Error Cluster From Error Code.vi"("show call chain? (False)"=TRUE, "error in (no error)"=w405, "error message (\"\")"=w406, "error code (0)"=w407) -> ()  [unwired: 5 in, 1 out]
        n112 = call <vilib>:"Add State(s) to Queue__JKI_lib_State_Machine.vi"("State(s) in (\"\")"=w410) -> ("States Out"=w409:string)  [unwired: 14 in]
      }
      frame "Target Buzy Error" {
        w422 = 42 items=["No error", "Argument error", "Memory is full", "Out of zone", "End of file", "File already open", "Generic file I/O error", "File not found", "File permission error", "Disk is full", "Duplicate path", "Too many files open", "System feature not enabled", "Resource file not found", "Cannot add resource", "Resource not found", "Image not found", "Image memory error", "Pen does not exist", "Config type invalid", "Config token not found", "Config parse error", "Config memory error", "Bad external code format", "Bad external code offset", "External code not present", "Null window", "Destroy window error", "Null menu", "Print aborted", "Bad print record", "Print driver error", "Windows error during printing", "Memory error during printing", "Print dialog error", "Generic print error", "Invalid device refnum", "Device not found", "Device parameter error", "Device unit error", "Cannot open device", "Device call aborted", "Generic error", "Cancelled by user", "Object ID too low", "Object ID too high", "Object not in heap", "Unknown heap", "Unknown object (invalid DefProc)", "Unknown object (DefProc not in table)", "Message out of range", "Invalid (null) method", "Unknown message", "Manager call not supported", "Bad address", "Network operation in progress", "Network operation timed out", "Connection is busy", "Network attribute not supported", "Network error", "Address in use", "System out of memory", "Connection aborted", "Connection refused", "Not connected", "Already connected", "Connection closed", "Initialization error (interapplication manager)", "Bad occurrence", "Wait on unbound occurrence handler", "Occurrence queue overflow", "Datalog type conflict", "Unused", "Unrecognized type (interapplication manager)", "Memory corrupt", "Failed to make temporary DLL", "Old CIN version", "Drag socket not found", "Failed to load drop-object", "Failed to register OLE object", "Failed to release OLE object", "Format specifier type mismatch", "Unknown format specifier", "Too few format specifiers", "Too many format specifiers", "Scan failed", "Newer CIN version", "Error converting to variant", "Runtime menu error", "Password tampered", "Variant attribute not found", "Incompatible variant data type", "Event data is not available", "Event Store is not present", "Occurrence is not found", "Event Queue is not created", "Event info is not available", "Refnum passed is NULL", "Error retrieving Class GUID", "Error retrieving CoClass GUID", "Error retrieving TypeLib GUID.", "Bad built application magic bytes.", "Specific driver is different from the specific driver associated with the Logical Name.", "There is no session opened to the class driver.", "Max Error", "MAX - Error with config objects", "MAX - Error loading configuration", "MAX - Group not supported"]
        # "Handle target buzy error here.\nWhen this JKISM try to communicate with a buzy target, this JKISM goes into this case."
        # "Handle mistyped state name (developer tool)"
        n113 = Format Into String(format string="Software Exception: Target is buzy now \"%s\"." ("message"), error in=w418, w414) -> (resulting string=w421:string, error out=w420:errorcluster)  [unwired: 1 in]
        n114 = call <vilib>:"Error Cluster From Error Code.vi"("show call chain? (False)"=TRUE, "error in (no error)"=w420, "error message (\"\")"=w421, "error code (0)"=w422) -> ("error out"=w419:errorcluster)  [unwired: 5 in]
        n115 = call <vilib>:"Add State(s) to Queue__JKI_lib_State_Machine.vi"("State(s) in (\"\")"=w413) -> ("States Out"=w417:string)  [unwired: 14 in]
      }
      frame "Target Timeout Error" {
        w433 = 42 items=["No error", "Argument error", "Memory is full", "Out of zone", "End of file", "File already open", "Generic file I/O error", "File not found", "File permission error", "Disk is full", "Duplicate path", "Too many files open", "System feature not enabled", "Resource file not found", "Cannot add resource", "Resource not found", "Image not found", "Image memory error", "Pen does not exist", "Config type invalid", "Config token not found", "Config parse error", "Config memory error", "Bad external code format", "Bad external code offset", "External code not present", "Null window", "Destroy window error", "Null menu", "Print aborted", "Bad print record", "Print driver error", "Windows error during printing", "Memory error during printing", "Print dialog error", "Generic print error", "Invalid device refnum", "Device not found", "Device parameter error", "Device unit error", "Cannot open device", "Device call aborted", "Generic error", "Cancelled by user", "Object ID too low", "Object ID too high", "Object not in heap", "Unknown heap", "Unknown object (invalid DefProc)", "Unknown object (DefProc not in table)", "Message out of range", "Invalid (null) method", "Unknown message", "Manager call not supported", "Bad address", "Network operation in progress", "Network operation timed out", "Connection is busy", "Network attribute not supported", "Network error", "Address in use", "System out of memory", "Connection aborted", "Connection refused", "Not connected", "Already connected", "Connection closed", "Initialization error (interapplication manager)", "Bad occurrence", "Wait on unbound occurrence handler", "Occurrence queue overflow", "Datalog type conflict", "Unused", "Unrecognized type (interapplication manager)", "Memory corrupt", "Failed to make temporary DLL", "Old CIN version", "Drag socket not found", "Failed to load drop-object", "Failed to register OLE object", "Failed to release OLE object", "Format specifier type mismatch", "Unknown format specifier", "Too few format specifiers", "Too many format specifiers", "Scan failed", "Newer CIN version", "Error converting to variant", "Runtime menu error", "Password tampered", "Variant attribute not found", "Incompatible variant data type", "Event data is not available", "Event Store is not present", "Occurrence is not found", "Event Queue is not created", "Event info is not available", "Refnum passed is NULL", "Error retrieving Class GUID", "Error retrieving CoClass GUID", "Error retrieving TypeLib GUID.", "Bad built application magic bytes.", "Specific driver is different from the specific driver associated with the Logical Name.", "There is no session opened to the class driver.", "Max Error", "MAX - Error with config objects", "MAX - Error loading configuration", "MAX - Group not supported"]
        # "Handle target timeout error here.\nWhen this JKISM could not get the sync-call response in time, this JKISM goes into this case."
        # "Handle mistyped state name (developer tool)"
        n116 = Format Into String(format string="Software Exception: Target could not finish the \"%s\" state in time." ("message"), error in=w429, w424) -> (resulting string=w432:string, error out=w431:errorcluster)  [unwired: 1 in]
        n117 = call <vilib>:"Error Cluster From Error Code.vi"("show call chain? (False)"=TRUE, "error in (no error)"=w431, "error message (\"\")"=w432, "error code (0)"=w433) -> ("error out"=w430:errorcluster)  [unwired: 5 in]
        n118 = call <vilib>:"Add State(s) to Queue__JKI_lib_State_Machine.vi"("State(s) in (\"\")"=w428) -> ("States Out"=w427:string)  [unwired: 14 in]
      }
      frame "Target Error" {
        w444 = 42 items=["No error", "Argument error", "Memory is full", "Out of zone", "End of file", "File already open", "Generic file I/O error", "File not found", "File permission error", "Disk is full", "Duplicate path", "Too many files open", "System feature not enabled", "Resource file not found", "Cannot add resource", "Resource not found", "Image not found", "Image memory error", "Pen does not exist", "Config type invalid", "Config token not found", "Config parse error", "Config memory error", "Bad external code format", "Bad external code offset", "External code not present", "Null window", "Destroy window error", "Null menu", "Print aborted", "Bad print record", "Print driver error", "Windows error during printing", "Memory error during printing", "Print dialog error", "Generic print error", "Invalid device refnum", "Device not found", "Device parameter error", "Device unit error", "Cannot open device", "Device call aborted", "Generic error", "Cancelled by user", "Object ID too low", "Object ID too high", "Object not in heap", "Unknown heap", "Unknown object (invalid DefProc)", "Unknown object (DefProc not in table)", "Message out of range", "Invalid (null) method", "Unknown message", "Manager call not supported", "Bad address", "Network operation in progress", "Network operation timed out", "Connection is busy", "Network attribute not supported", "Network error", "Address in use", "System out of memory", "Connection aborted", "Connection refused", "Not connected", "Already connected", "Connection closed", "Initialization error (interapplication manager)", "Bad occurrence", "Wait on unbound occurrence handler", "Occurrence queue overflow", "Datalog type conflict", "Unused", "Unrecognized type (interapplication manager)", "Memory corrupt", "Failed to make temporary DLL", "Old CIN version", "Drag socket not found", "Failed to load drop-object", "Failed to register OLE object", "Failed to release OLE object", "Format specifier type mismatch", "Unknown format specifier", "Too few format specifiers", "Too many format specifiers", "Scan failed", "Newer CIN version", "Error converting to variant", "Runtime menu error", "Password tampered", "Variant attribute not found", "Incompatible variant data type", "Event data is not available", "Event Store is not present", "Occurrence is not found", "Event Queue is not created", "Event info is not available", "Refnum passed is NULL", "Error retrieving Class GUID", "Error retrieving CoClass GUID", "Error retrieving TypeLib GUID.", "Bad built application magic bytes.", "Specific driver is different from the specific driver associated with the Logical Name.", "There is no session opened to the class driver.", "Max Error", "MAX - Error with config objects", "MAX - Error loading configuration", "MAX - Group not supported"]
        # "Handle target error here.\nWhen this JKISM try to communicate with an un-existed JKISM, this JKISM goes into this case."
        # "Handle mistyped state name (developer tool)"
        n119 = Format Into String(format string="Software Exception: Target \"%s\" does not exists." ("message"), error in=w440, w435) -> (resulting string=w443:string, error out=w442:errorcluster)  [unwired: 1 in]
        n120 = call <vilib>:"Add State(s) to Queue__JKI_lib_State_Machine.vi"("State(s) in (\"\")"=w439) -> ("States Out"=w438:string)  [unwired: 14 in]
        n121 = call <vilib>:"Error Cluster From Error Code.vi"("show call chain? (False)"=TRUE, "error in (no error)"=w442, "error message (\"\")"=w443, "error code (0)"=w444) -> ("error out"=w441:errorcluster)  [unwired: 5 in]
      }
      frame "Async Response", "Response" {
        # "Handle Async-call Response (\"Async Response\" for ->)"
        # "Handle Sync-call Response (\"Response\" for @)"
        # "After Message is excuted, JKISM+ goes to this state for recieve the response. \n    For Async Message(->), \"Async Response\" is used. This JKISM will goes to \"Async Message Posted\" immediately and recieve the \"Async Response\" after the callee finishes the message.\n    For Sync Message(@),  This JKISM will wait until the message is done and immidieatly goes to \"Response\""
      }
      frame "Async Message Posted" {
        # "Handle post action for async message (->)."
        # "After Async Message is posted (->), JKISM+ goes to this state for post-action. You can use Argument - State to tell which Async Message is called."
      }
      frame "Initialize Core Data" {
        # "Do not delete, rename, or modify this frame.\n(this is used to determine panel behavior on exit)"
        # "originally closed?"
        # "exe?"
        # "If panel starts closed or is an EXE, then close it when we exit"
        n122 = property class="VI"() -> ("FP.State"=w454:T1)  [unwired: 2 in, 2 out]
        n123 = property class="App"() -> ("App.Kind"=w460:T2)  [unwired: 2 in, 2 out]
        n124 = control-ref of="Current VI Reference"() -> (w455:refnum<vi>)
        n125 = Equal?(x=w454, y=T1."Closed" ("Front Panel Window:State")) -> (x = y?=w452:bool)
        n126 = Equal?(x=w460, y=T2."Run Time System" ("Application:Kind")) -> (x = y?=w458:bool)
        n127 = Or(x=w452, y=w458) -> (x .or. y?=w456:bool)
        n128 = Bundle By Name(cluster=w457, "Core.Current VI Reference"=w455, "Core.Close Panel on Exit?"=w456) -> (w462:T5)
        n129 = call <vilib>:"Add State(s) to Queue__JKI_lib_State_Machine.vi"("State(s) in (\"\")"=w464) -> ("States Out"=w463:string)  [unwired: 14 in]
      }
      frame "Exit" {
        # "Do not put any code in this frame.\n(No errors that occur here will be handled.)"
        n130 = call <vilib>:"Add State(s) to Queue__JKI_lib_State_Machine.vi"("State(s) in (\"\")"=w469) -> ("States Out"=w468:string)  [unwired: 14 in]
      }
      frame "---------- Data ----------" {
        # "Do not put any code in this frame.\n(It is a separator no-op. You can make a copy of this frame to create a new Data frame)"
        n131 = call <vilib>:"Add State(s) to Queue__JKI_lib_State_Machine.vi"("State(s) in (\"\")"=w473) -> ("States Out"=w472:string)  [unwired: 14 in]
      }
      frame "Data: Initialize" {
        w474 = T4 {"Current VI Reference"=refnum, "Close Panel on Exit?"=FALSE}  # Core
        w476 = TRUE  # Your Boolean data
        w475 = ""  # Your string data
        # "do not delete - used by framework"
        # "Expand Bundle to add new data elements to shift register data."
        # "Add new data here."
        # "Initialize the shift-register data, here.\n(data names are defined by what you wire into the bundle function)"
        n132 = Bundle("Core"=w474, "Your Boolean data"=w476, "Your string data"=w475) -> (w478:T5)  [unwired: 1 in]
        n133 = call <vilib>:"Add State(s) to Queue__JKI_lib_State_Machine.vi"("State(s) in (\"\")"=w480) -> ("States Out"=w479:string)  [unwired: 14 in]
      }
      frame "Data: Cleanup" {
        # "Cleanup any data and references, here.\n(this is called automatically, by the Macro: Exit)"
        n134 = Unbundle By Name(w481) -> ("Core.Current VI Reference"=w484:refnum<vi>)
        n135 = Close Reference(reference=w484, error in (no error)=w483) -> (error out=w482:errorcluster)
        n136 = call <vilib>:"Add State(s) to Queue__JKI_lib_State_Machine.vi"("State(s) in (\"\")"=w486) -> ("States Out"=w485:string)  [unwired: 14 in]
      }
      frame "---------- Macro ----------" {
        # "Do not put any code in this frame.\n(It is a separator no-op. You can make a copy of this frame to create a new Macro frame)"
        n137 = call <vilib>:"Add State(s) to Queue__JKI_lib_State_Machine.vi"("State(s) in (\"\")"=w490) -> ("States Out"=w489:string)  [unwired: 14 in]
      }
      frame "Macro: Initialize" {
        # "Initialization Macro\n(This is called once, when the VI starts)"
        n138 = call <vilib>:"Add State(s) to Queue__JKI_lib_State_Machine.vi"("State(s) in Front (\"\")"="Data: Initialize\nInitialize Core Data", "State(s) in (\"\")"=w495) -> ("States Out"=w494:string)  [unwired: 13 in]
      }
      frame "Macro: Exit" {
        # "Exit Macro\n(This is called once, when the VI exits)"
        n139 = call <vilib>:"Add State(s) to Queue__JKI_lib_State_Machine.vi"("State(s) in Front (\"\")"="Data: Cleanup\nExit", "State(s) in (\"\")"=w500) -> ("States Out"=w499:string)  [unwired: 13 in]
      }
      frame "---------- API ----------" {
        # "Do not put any code in this frame.\n(It is a separator no-op. This category is recommanded to use for external API)"
      }
      frame "API: API1" {
        # "If you need to tell who triggered this state , use this string. If it's this case itself, this string is \"\"."
        # "Deal with the parameter if any"
        # "Connect this to return the response of your API"
        # "Copy/Rename this case for your own API"
      }
      frame "API: API2" {
        # "unpack HexStr  to Variant\nif complex parameter is needed."
        # "Copy/Rename this case for your own API"
        n140 = call "JKISM++ Convert HexStr to Data.vi"("HEX String"=w509) -> ()  [unwired: 8 in, 1 out]
        n141 = disable-structure shown="Enabled" {
          disable-tunnel: [w513 "API2 Response"] -> w508
          frame Disabled {
            # "pack variant to hexstr \nif complex response is needed."
            # "complex Response"
            n142 = call "JKISM++ Convert Data to HexStr.vi"() -> ("HEX String (0-9,A-F)"=w513:string)  [unwired: 9 in]
          }
          frame Enabled {
          }
        }
      }
      frame "---------- DoSth ----------" {
        # "Template Separator\n(You can make a copy of, or modify, this frame)"
        n143 = call <vilib>:"Add State(s) to Queue__JKI_lib_State_Machine.vi"("State(s) in (\"\")"=w518) -> ("States Out"=w517:string)  [unwired: 14 in]
      }
      frame "SM: Step2" {
        n144 = Wait (ms)(milliseconds to wait=u32 500) -> ()  [unwired: 1 out]
        n145 = call <vilib>:"Add State(s) to Queue__JKI_lib_State_Machine.vi"("State(s) in (\"\")"=w524) -> ("States Out"=w523:string)  [unwired: 14 in]
      }
      frame "SM: Step4" {
        n146 = Wait (ms)(milliseconds to wait=u32 500) -> ()  [unwired: 1 out]
        n147 = call <vilib>:"Add State(s) to Queue__JKI_lib_State_Machine.vi"("State(s) in (\"\")"=w530) -> ("States Out"=w529:string)  [unwired: 14 in]
      }
    }
  }
